vi "Chart[Template].Clear.vi"(8 "error in (no error)":errorcluster, 11 "Chart":refnum<class "Chart.lvclass">) -> (0 "error out":errorcluster, 3 "Chart out":refnum<class "Chart.lvclass">)   [LabVIEW 2019, in "Chart.lvclass"]
doc: "---------------------------------------------------------------\nJKI State Machine Objects™\nhttp://jki.net/state-machine-objects/\nCopyright (C) 2005-2015, JKI <info@jki.net>\nALL RIGHTS RESERVEDJKI State Machine Objects (SMO) 1.0.0.5\nJKI - JKI\nCopyright (c) 2016, JKI"
uses:
  Chart.lvclass
  Chart.lvclass/Chart.ctl
panel:
  # "For instructions on how to use the JKI State Machine Objects, examples and video tutorials, visit:\nhttp://jki.net/state-machine-objects/\n\nJKI State Machine Objects™\nhttp://jki.net/state-machine-objects/\nCopyright (C) 2005-2015, JKI <info@jki.net>\nALL RIGHTS RESERVED"
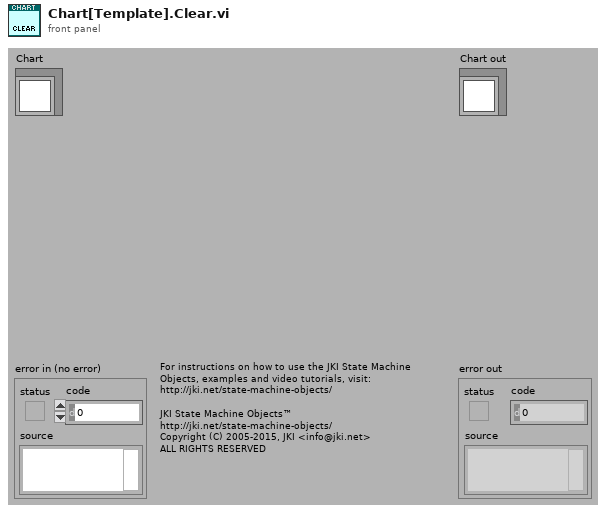
[diagram p1: front panel]
types:
  T1 = typedef "Chart.lvclass/PublicEvents--Cluster.ctl" = cluster{"Chart cleared":refnum<user-event>}
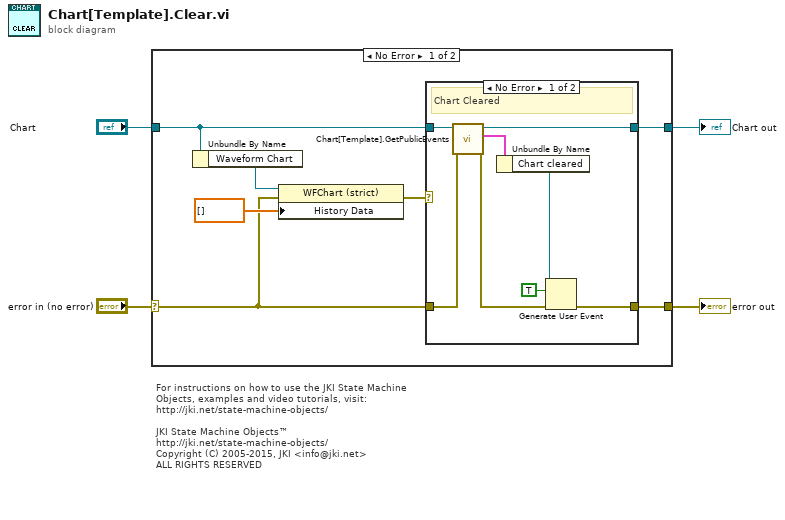
[diagram p0: block diagram]
diagram:
  # "For instructions on how to use the JKI State Machine Objects, examples and video tutorials, visit:\nhttp://jki.net/state-machine-objects/\n\nJKI State Machine Objects™\nhttp://jki.net/state-machine-objects/\nCopyright (C) 2005-2015, JKI <info@jki.net>\nALL RIGHTS RESERVED"
  n1 = case shown="No Error" "error in (no error)" {
    selector: "error in (no error)" -> [w5 w22]
    tunnel: "Chart" -> [w9 w23]
    tunnel: [w11 w22] -> w3
    tunnel: [w10 w23] -> w2
    frame No Error {
      n2 = Unbundle By Name(w9) -> ("Waveform Chart"=w8:refnum<vi>)
      n3 = property class="WFChart (strict)"(reference=w8, error in=w5, "History Data"=dbl[] []) -> (error out=w6:errorcluster)  [unwired: 1 out]
      n4 = case shown="No Error" w6 {
        tunnel: w5 -> [w17 w20]
        tunnel: [w14 w20] -> w11
        tunnel: w9 -> [w19 w21]
        tunnel: [w18 w21] -> w10
        frame No Error {
          # "Chart Cleared"
          n5 = call "Chart[Template].GetPublicEvents.vi"("error in (no error)"=w17, "Chart"=w19) -> ("error out"=w15:errorcluster, "Chart[Template] Public Events"=w16:T1, "Chart out"=w18:refnum<class "Chart.lvclass">)  [unwired: 7 in]
          n6 = Unbundle By Name(w16) -> ("Chart cleared"=w12:refnum<user-event>)
          n7 = Generate User Event(user event=w12, event data cluster=TRUE ("event data"), error in=w15) -> (error out=w14:errorcluster)  [unwired: 1 in, 1 out]
        }
        frame Error {
          # "Chart was not cleared"
        }
      }
    }
    frame Error {
    }
  }
  "error out" <- w3
  "Chart out" <- w2
